vi "CheckValidReference.vi"(7 "check all queues? (F)":bool, 8 "error in":errorcluster, 11 "message ref in":refnum<class "CLM_PriorityLocalMessage.lvclass">) -> (0 "error out":errorcluster, 2 "valid?":bool, 3 "message ref out":refnum<class "CLM_PriorityLocalMessage.lvclass">)   [LabVIEW 2013, in "CLM_PriorityLocalMessage.lvclass"]
uses:
  CLM_PriorityLocalMessage.lvclass
  CLM_PriorityLocalMessage.lvclass/CLM_PriorityLocalMessage.ctl
  LocalMessage_Queue/CLM_LocalMessage_Queue.lvclass/CLM_LocalMessage_Queue.ctl
  LocalMessage_Queue/CLM_LocalMessage_Queue.lvclass
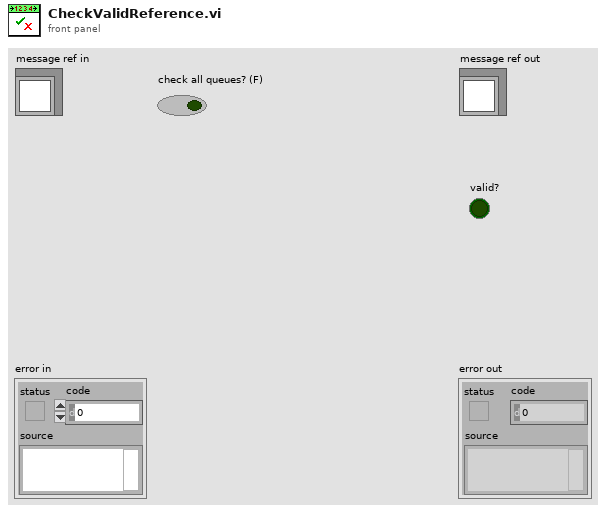
[diagram p1: front panel]
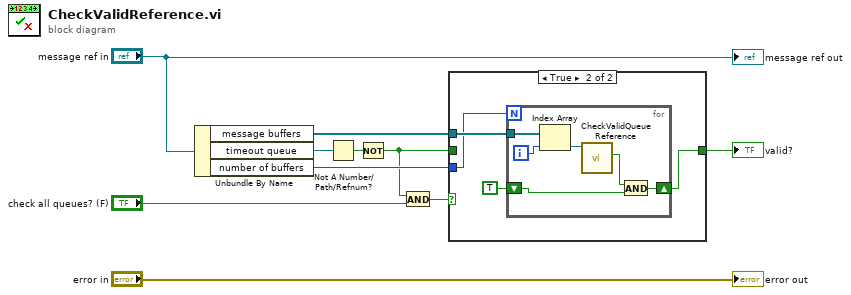
[diagram p0: block diagram]
diagram:
  n1 = Unbundle By Name("message ref in") -> ("message buffers"=w5:refnum<class "CLM_LocalMessage_Queue.lvclass">[], "timeout queue"=w3:refnum<queue>, "number of buffers"=w6:i32)
  n2 = Not A Number/Path/Refnum?(number/path/refnum=w3) -> (NaN/Path/Refnum?=w4:bool)
  n3 = Not(x=w4) -> (.not. x?=w2:bool)
  n4 = And(x=w2, y="check all queues? (F)") -> (x .and. y?=w1:bool)
  n5 = case shown="True" w1 {
    tunnel: w6 -> [_ w14]
    tunnel: w5 -> [_ w15]
    tunnel: w2 -> [w11 _]
    tunnel: [w11 w13] -> w7
    frame False {
    }
    frame True {
      n6 = for {
        N: w14 -> [_]
        tunnel: w15 -> [w21]
        shift-right: [w17] -> w13
        shift-left: TRUE -> [w16]
        i -> [w20]
        n7 = Index Array(array=w21, index=w20) -> (element=w19:refnum<class "CLM_LocalMessage_Queue.lvclass">)
        n8 = call "CheckValidQueueReference.vi"("message ref in"=w19) -> ("valid?"=w18:bool)  [unwired: 8 in, 2 out]
        n9 = And(x=w18, y=w16) -> (x .and. y?=w17:bool)
      }
    }
  }
  "valid?" <- w7
  "error out" <- "error in"
  "message ref out" <- "message ref in"
